vi "Get Project Ref and Name.vi"(11 "Project Name":string) -> (1 "Found?":bool, 3 "Project Refnum":refnum<vi>)   [LabVIEW 2020, in "Panter Dashboard.lvlib"]
uses:
  Panter Dashboard.lvlib
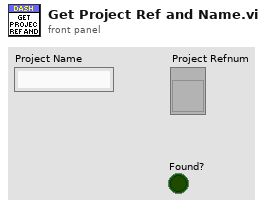
[diagram p1: front panel]
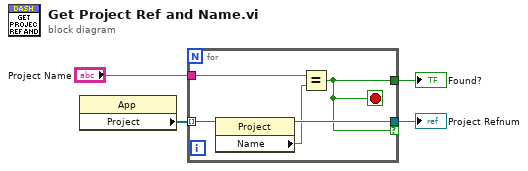
[diagram p0: block diagram]
diagram:
  n1 = property class="App"() -> ("Project"=w3:refnum<vi>[])  [unwired: 2 in, 2 out]
  n2 = for {
    tunnel: w3 -> [w9] mode=indexing
    tunnel: "Project Name" -> [w6]
    tunnel: [w8] -> w2 if=w5
    tunnel: [w5] -> w1
    stop <- w5 stop-if-true
    n3 = property class="Project"(reference=w9) -> (reference out=w8:refnum<vi>, "Name"=w7:string)  [unwired: 1 in, 1 out]
    n4 = Equal?(x=w6, y=w7) -> (x = y?=w5:bool)
  }
  "Project Refnum" <- w2
  "Found?" <- w1
